vi "Create AO Channel.vi"(8 "error in (no error)":errorcluster, 11 "AO Channel Setting":T1) -> (0 "error out":errorcluster, 3 "AO Task":refnum<k21>)   [LabVIEW 2023, in "DAQ Hardware.lvlib"]
uses:
  DAQ Hardware.lvlib
  AO Channel Setting.ctl
  <vilib>/DAQmx/create/channels.llb/DAQmx Create Channel (AO-Voltage-Basic).vi
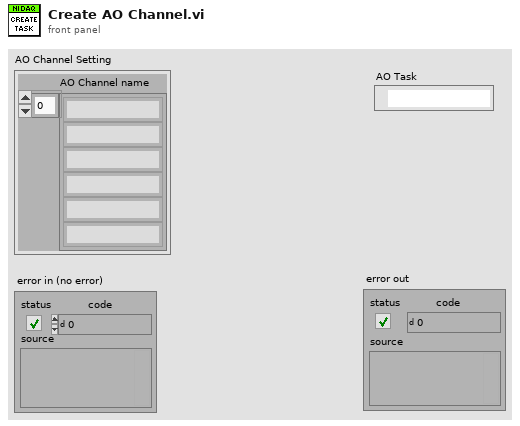
[diagram p1: front panel]
types:
  T1 = typedef "DAQ Hardware.lvlib/AO Channel Setting.ctl" = cluster{"AO Channel name":string[]}
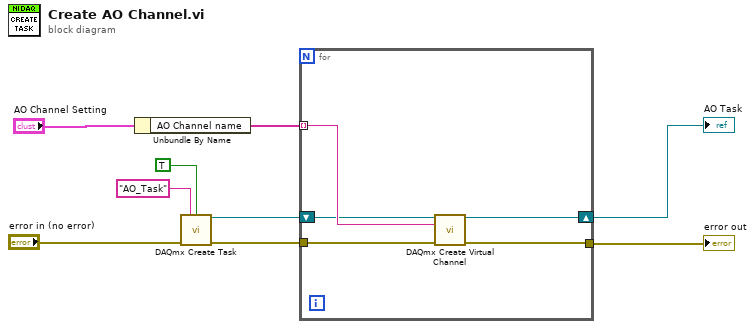
[diagram p0: block diagram]
diagram:
  n1 = Unbundle By Name("AO Channel Setting") -> ("AO Channel name"=w7:string[])
  n2 = call <vilib>:"DAQmx Create Task.vi"("new task name"="AO_Task", "auto cleanup"=TRUE, "error in"="error in (no error)") -> ("task out"=w2:refnum<k21>, "error out"=w3:errorcluster)  [unwired: 11 in]
  n3 = for {
    tunnel: w3 -> [w13]
    tunnel: w7 -> [w14] mode=indexing
    tunnel: [w12] -> w9
    shift-right: [w10] -> w1
    shift-left: w2 -> [w11]
    n4 = call-poly <vilib>:"DAQmx Create Virtual Channel.vi"("task in"=w11, "physical channels"=w14, "error in"=w13) -> ("task out"=w10:refnum<k21>, "error out"=w12:errorcluster)  [unwired: 11 in]
  }
  "error out" <- w9
  "AO Task" <- w1
